vi "Add Component Dependencies.vi"(8 "error in (no error)":errorcluster, 11 "Device Item Ref in":T1 format="%.0x") -> (0 "error out":errorcluster, 2 "component names":string[](array[string]), 3 "Device Ref out":T1 format="%.0x")   [LabVIEW 2017, in "DSF System Explorer.lvlib"]
uses:
  DSF System Explorer.lvlib
  <vilib>/NI Veristand/Custom Device API/Custom Device Item Ref.ctl
  <vilib>/NI Veristand/Custom Device API/Set Item Property (Path).vi
  <vilib>/NI VeriStand/Custom Device API/Custom Device API.lvlib
  Shared/DSF Shared.lvlib
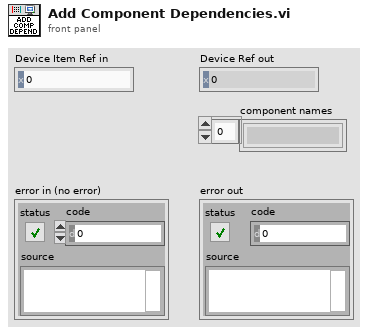
[diagram p1: front panel]
types:
  T1 = typedef "Custom Device API.lvlib/Custom Device Item Ref.ctl" = u64
  T2 = typedef "Custom Device API.lvlib/Custom Device Target Type.ctl" = enum16{"PharLap", "VxWorks", "Windows", "Linux_32_ARM", "Linux_x64"}
  T3 = typedef "Custom Device API.lvlib/Custom Device File Dependency.ctl" = cluster{"Source":T4, "RT Destination":path, "ForceDownload?":bool, "SupportedTarget":T6, "Version":string}
  T4 = typedef "Custom Device API.lvlib/Path Specification.ctl" = cluster{"Path":path, "Type":T5}
  T5 = typedef "Custom Device API.lvlib/Path Type.ctl" = enum16{"Absolute", "To Base", "To Common Data Dir", "To Application Data Dir"}
  T6 = typedef "Custom Device API.lvlib/Custom Device Supported Target.ctl" = enum16{"All", "PharLap", "VxWorks", "Windows", "Linux_32_ARM", "Linux_x64", "PharLap & Windows", "PharLap & VxWorks", "VxWorks & Windows"}
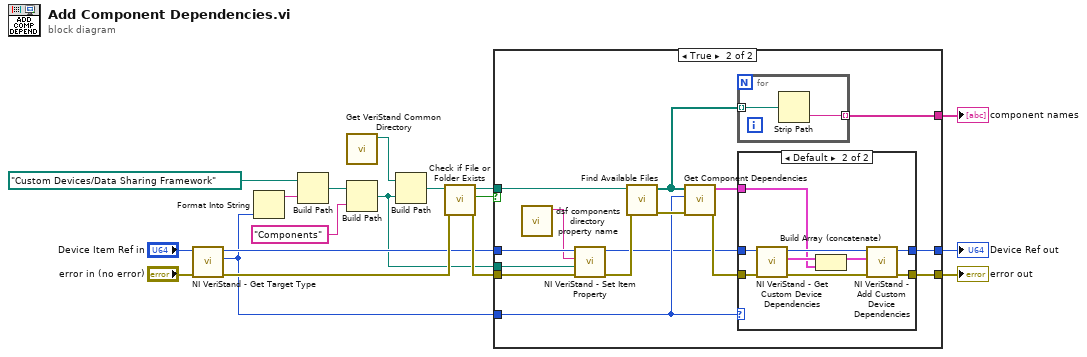
[diagram p0: block diagram]
diagram:
  n1 = call <vilib>:"NI VeriStand - Get Target Type.vi"("error in (no error)"="error in (no error)", "Item Ref in"="Device Item Ref in") -> ("error out"=w10:errorcluster, "Target Type"=w2:T2, "Item Ref out"=w8:T1)  [unwired: 7 in]
  n2 = Format Into String(w2) -> (resulting string=w1:string)  [unwired: 3 in, 1 out]
  n3 = Build Path(base path=path "Custom Devices/Data Sharing Framework", name or relative path=w1) -> (appended path=w15:path)
  n4 = call "Get VeriStand Common Directory.vi"() -> ("common directory"=w17:path)  [unwired: 11 in]
  n5 = Build Path(base path=w15, name or relative path="Components") -> (appended path=w3:path)
  n6 = Build Path(base path=w17, name or relative path=w3) -> (appended path=w4:path)
  n7 = call <vilib>:"Check if File or Folder Exists.vi"("error in (no error)"=w10, "path"=w4) -> ("error out"=w9:errorcluster, "file or folder exists?"=w7:bool, "dup path"=w11:path)  [unwired: 7 in]
  n8 = case shown="True" w7 {
    tunnel: [w19 w35] -> w18
    tunnel: [w20 w34] -> w6
    tunnel: [_ w29] -> w14
    tunnel: w8 -> [w19 w28]
    tunnel: w2 -> [_ w27]
    tunnel: w11 -> [_ w23]
    tunnel: w9 -> [w20 w22]
    tunnel: w3 -> [_ w21]
    frame False {
    }
    frame True {
      n9 = call "dsf components directory property name.vi"() -> ("components directory property name"=w24:string)  [unwired: 11 in]
      n10 = call-poly <vilib>:"NI VeriStand - Set Item Property.vi"("error in (no error)"=w22, "Value"=w21, "Property Name"=w24, "Item Ref in"=w28) -> ("error out"=w26:errorcluster, "Item Ref out"=w25:T1)  [unwired: 5 in, 1 out]
      n11 = call "Find Available Files.vi"("error in (no error)"=w26, "components directory"=w23) -> ("error out"=w31:errorcluster, "paths"=w30:path[])  [unwired: 8 in]
      n12 = call "Get Component Dependencies.vi"("error in (no error)"=w31, "Target Type"=w27, "component paths"=w30) -> ("error out"=w33:errorcluster, "component dependencies"=w32:T3[])  [unwired: 7 in]
      n13 = for {
        tunnel: w30 -> [w37] mode=indexing
        tunnel: [w36] -> w29 mode=indexing
        n14 = Strip Path(path=w37) -> (name=w36:string)  [unwired: 1 out]
      }
      n15 = case shown="Default" w27 {
        tunnel: w32 -> [_ w41]
        tunnel: w33 -> [w39 w47]
        tunnel: w25 -> [w38 w48]
        tunnel: [w39 w42] -> w34
        tunnel: [w38 w40] -> w35
        frame "Windows" {
          # "Don't add dependencies for Windows."
        }
        frame Default {
          n16 = call <vilib>:"NI VeriStand - Get Custom Device Dependencies.vi"("error in (no error)"=w47, "Device Ref in"=w48) -> ("error out"=w45:errorcluster, "Dependencies"=w46:T3[], "Device Ref out"=w43:T1)  [unwired: 7 in]
          n17 = Build Array (concatenate)(w46, w41) -> (w44:T3[])
          n18 = call <vilib>:"NI VeriStand - Add Custom Device Dependencies.vi"("error in (no error)"=w45, "Dependencies"=w44, "Device Ref in"=w43) -> ("error out"=w42:errorcluster, "Device Ref out"=w40:T1)  [unwired: 7 in]
        }
      }
    }
  }
  "Device Ref out" <- w18
  "error out" <- w6
  "component names" <- w14
